vi "ProgramPixelReg.vi"(5 "Chip ID list":u32[](array[numeric]) format="%x", 7 "Pixel Register":u32[](array[numeric])=[671965161, 384, 671965161, 384, 671965161, 384, 671965161, 384, 671965161, 384, 671965161, 384, 671965161, 384, 671965161, 384, 671965161, 384, 671965161, 384, 671965161, 384, 671965161, 384, 671965161, 384, 671965161, 384, 671965161, 384, 671965161, 384, 671965161, 384, 671965161, 384, 671965161, 384, 671965161, 384, 671965161, 384, 671965161, 384, 671965161, 384, 671965161, 384, 671965161, 384, 671965161, 384, 671965161, 384, 671965161, 384, 671965161, 384, 671965161, 384, 671965161, 384, 671965161, 384, 671965161, 384, 671965161, 384, 671965161, 384, 671965161, 384, 671965161, 384, 671965161, 384, 671965161, 384, 671965161, 384, 671965161, 384, 671965161, 384, 671965161, 384, 671965161, 384, 671965161, 384, 671965161, 384, 671965161, 384, 671965161, 384, 671965161, 384, 671965161, 384, 671965161, 384, 671965161, 384, 671965161, 384, 671965161, 384, 671965161, 384, 671965161, 384, 671965161, 384, 671965161, 384, 671965161, 384, 671965161, 384, 671965161, 384, 671965161, 384, 671965161, 384, 671965161, 384, 671965161, 384, 671965161, 384, 671965161, 384, 671965161, 384, 671965161, 384, 671965161, 384, 671965161, 384, 671965161, 384, 671965161, 384, 671965161, 384, 671965161, 384, 671965161, 384, 671965161, 384, 671965161, 384, 671965161, 384, 671965161, 384, 671965161, 384, 671965161, 384, 671965161, 384, 671965161, 384, 671965161, 384, 671965161, 384, 671965161, 384, 671965161, 384, 671965161, 384, 671965161, 384, 671965161, 384, 671965161, 384, 671965161, 384, 671965161, 384, 671965161, 384, 671965161, 384, 671965161, 384, 671965161, 384, 671965161, 384, 671965161, 384] format="%x", 8 "error in (no error)":errorcluster, 9 "ChipID":u32=65535 format="%x", 10 "LayerID":u32=65535 format="%x", 11 "connection ID":refnum<k5>) -> (0 "error out":errorcluster, 1 "OK?":bool, 2 "PixelReg programmed":u32[](array[numeric]), 3 "connection ID out":refnum<k5>, 4 "Program done":string[](array[string]))   [LabVIEW 2015, in "VIPM2.lvlib"]
uses:
  VIPM2.lvlib
panel:
  out "Ready to receive data":string
  # "Program Pixel Register"
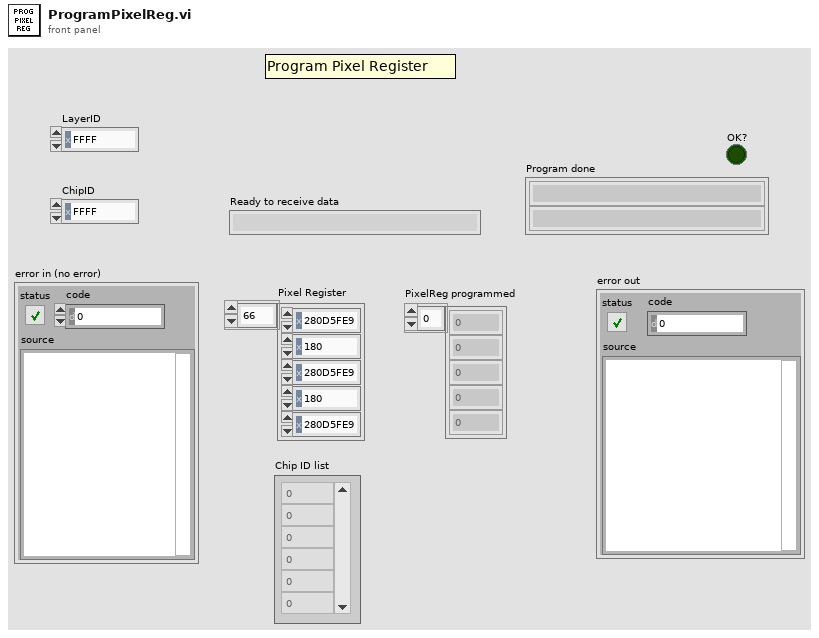
[diagram p1: front panel]
types:
  T1 = enum16{"Standard", "Buffered", "CRLF", "Immediate"}
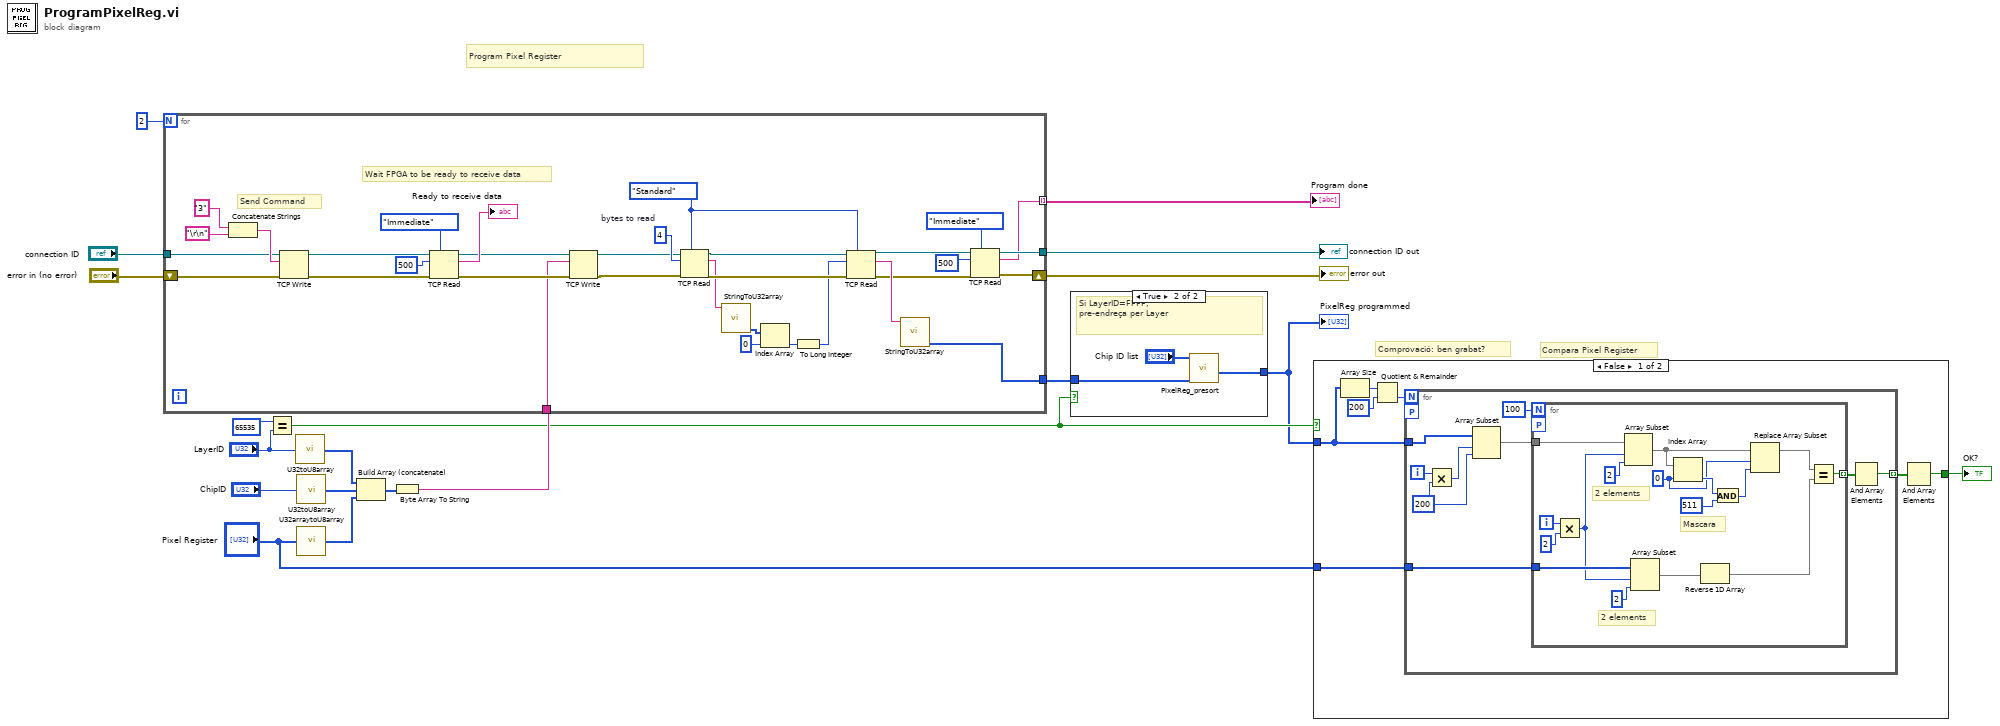
[diagram p0: block diagram]
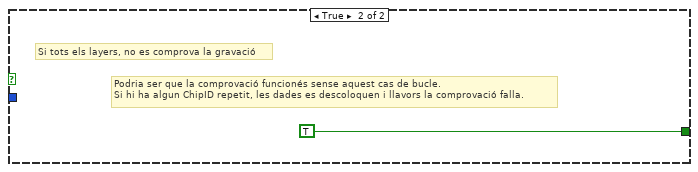
[diagram p3: hidden frame]
diagram:
  # "Compara Pixel Register"
  # "Comprovació: ben grabat?"
  # "Program Pixel Register"
  n1 = Equal?(x=u32 65535 ("LayerID 2"), y="LayerID") -> (x = y?=w3:bool)
  n2 = call "U32toU8array.vi"("x"="LayerID") -> ("ArrayU8"=w15:u8[])
  n3 = call "U32toU8array.vi"("x"="ChipID") -> ("ArrayU8"=w14:u8[])
  n4 = call "U32arraytoU8array.vi"("ArrayU32"="Pixel Register") -> ("ArrayU8"=w13:u8[])
  n5 = Build Array (concatenate)(w15, w14, w13) -> (w16:u8[])
  n6 = Byte Array To String(unsigned byte array=w16) -> (string=w12:string)
  n7 = for {
    N: 2 -> [_]
    tunnel: "connection ID" -> [w49]
    tunnel: [w41] -> w18
    tunnel: [w40] -> w9 mode=indexing
    tunnel: w12 -> [w37]
    shift-right: [w23] -> w10
    shift-left: "error in (no error)" -> [w24]
    tunnel: [w22] -> w2
    w32 = 4  # bytes to read
    w33 = T1."Standard" ("mode (standard)")
    # "Wait FPGA to be ready to receive data"
    # "Send Command"
    n8 = Concatenate Strings("3" ("string"), "\r\n") -> (w50:string)
    n9 = TCP Write(connection ID=w49, data in=w50, error in (no error)=w24) -> (connection ID out=w45:refnum<k5>, error out=w44:errorcluster)  [unwired: 1 in, 1 out]
    n10 = TCP Read(connection ID=w45, bytes to read=500, error in (no error)=w44, 7:T1."Immediate" ("mode (standard)")) -> (connection ID out=w39:refnum<k5>, data out=→"Ready to receive data":string, error out=w38:errorcluster)  [unwired: 1 in]
    n11 = TCP Write(connection ID=w39, data in=w37, error in (no error)=w38) -> (connection ID out=w30:refnum<k5>, error out=w31:errorcluster)  [unwired: 1 in, 1 out]
    n12 = TCP Read(connection ID=w30, bytes to read=w32, error in (no error)=w31, 7:w33) -> (connection ID out=w36:refnum<k5>, data out=w29:string, error out=w35:errorcluster)  [unwired: 1 in]
    n13 = call "StringToU32array.vi"("String"=w29) -> ("U32array"=w28:u32[])  [unwired: 2 out]
    n14 = Index Array(array=w28, index=0) -> (element=w21:u32)
    n15 = To Long Integer(number=w21) -> (32bit integer=w20:i32)
    n16 = TCP Read(connection ID=w36, bytes to read=w20, error in (no error)=w35, 7:w33) -> (connection ID out=w26:refnum<k5>, data out=w27:string, error out=w25:errorcluster)  [unwired: 1 in]
    n17 = call "StringToU32array.vi"("String"=w27) -> ("U32array"=w22:u32[])  [unwired: 2 out]
    n18 = TCP Read(connection ID=w26, bytes to read=500, error in (no error)=w25, 7:T1."Immediate" ("mode (standard)")) -> (connection ID out=w41:refnum<k5>, data out=w40:string, error out=w23:errorcluster)  [unwired: 1 in]
  }
  "connection ID out" <- w18
  "error out" <- w10
  "Program done" <- w9
  n19 = case shown="True" w3 {
    tunnel: w2 -> [w53 w56]
    tunnel: [w53 w55] -> w1
    frame False {
    }
    frame True {
      # "Si LayerID=FFFF,\npre-endreça per Layer"
      n20 = call "PixelReg_presort.vi"("EQ Data and Report"=w56, "Chip ID list"="Chip ID list") -> ("EQ Data and Report out"=w55:u32[])  [unwired: 9 in]
    }
  }
  "PixelReg programmed" <- w1
  n21 = case shown="False" w3 {
    tunnel: w1 -> [w58 _]
    tunnel: "Pixel Register" -> [w63 _]
    tunnel: [w61 TRUE] -> w6
    frame False {
      n22 = Array Size(array=w58) -> (size(s)=w59:i32)
      n23 = Quotient & Remainder(x=w59, y=200) -> (floor(x/y)=w60:i32)  [unwired: 1 out]
      n24 = for {
        N: w60 -> [_]
        tunnel: w58 -> [w67]
        tunnel: w63 -> [w72]
        tunnel: [w70] -> w62 mode=indexing
        workers-P: _ -> [_]
        i -> [w66]
        w64 = 200 ("y")
        n25 = Multiply(x=w66, y=w64) -> (x*y=w65:i32)
        n26 = Array Subset(array=w67, index=w65, length=w64) -> (w68:u32[])
        n27 = for {
          N: 100 -> [_]
          tunnel: [w85] -> w69 mode=indexing
          tunnel: w68 -> [w79]
          tunnel: w72 -> [w78]
          workers-P: _ -> [_]
          i -> [w77]
          w81 = 0 ("index")
          # "2 elements"
          # "2 elements"
          # "Mascara"
          n28 = Multiply(x=w77, y=2) -> (x*y=w75:i32)
          n29 = Array Subset "Array Subset"(array=w79, index=w75, length=2) -> (w87:u32[])
          n30 = Array Subset "Array Subset"(array=w78, index=w75, length=2) -> (w74:u32[])
          n31 = Index Array(array=w87, index=w81) -> (element=w84:u32)
          n32 = Reverse 1D Array(array=w74) -> (reversed array=w73:u32[])
          n33 = And(x=w84, y=u32 511) -> (x .and. y?=w82:u32)
          n34 = Replace Array Subset "Replace Array Subset"(array=w87, new element=w82, index=w81) -> (w86:u32[])
          n35 = Equal?(x=w86, y=w73) -> (x = y?=w85:bool)
        }
        n36 = And Array Elements(Boolean array=w69) -> (logical AND=w70:bool)
      }
      n37 = And Array Elements(Boolean array=w62) -> (logical AND=w61:bool)
    }
    frame True {
      # "Podria ser que la comprovació funcionés sense aquest cas de bucle.\nSi hi ha algun ChipID repetit, les dades es descoloquen i llavors la comprovació falla."
      # "Si tots els layers, no es comprova la gravació"
    }
  }
  "OK?" <- w6
